vi "StringToHex.vi"(8 "error in (no error)":errorcluster caption="错误输入（无错误）", 11 "String_Hex":string="55AA001200050104110000000000000000000000000000000000000000000000") -> (0 "error out":errorcluster caption="错误输出", 2 "Hex":string)   [LabVIEW 2015]
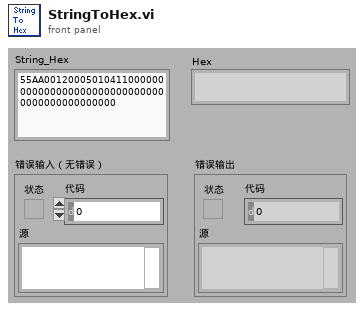
[diagram p1: front panel]
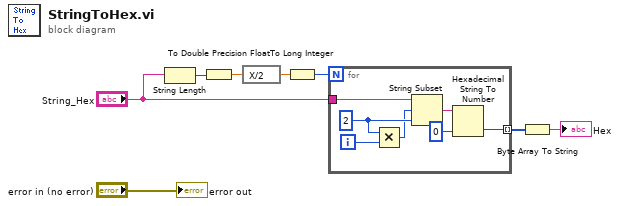
[diagram p0: block diagram]
diagram:
  n1 = String Length(string="String_Hex") -> (length=w8:i32)
  n2 = To Double Precision Float(number=w8) -> (double precision float=w7:dbl)
  n3 = expression code="X/2"(w7) -> (w6:dbl)
  n4 = To Long Integer(number=w6) -> (32bit integer=w5:i32)
  n5 = for {
    N: w5 -> [_]
    tunnel: "String_Hex" -> [w15]
    tunnel: [w10] -> w4 mode=indexing
    i -> [w14]
    w13 = 2 ("长度（剩余）")
    n6 = Multiply(x=w13, y=w14) -> (x*y=w12:i32)
    n7 = String Subset(string=w15, offset (0)=w12, length (rest)=w13) -> (substring=w9:string)
    n8 = Hexadecimal String To Number(string=w9, default (0uL)=u8 0 ("默认(0 U32)")) -> (number=w10:u8)  [unwired: 2 out]
  }
  n9 = Byte Array To String(unsigned byte array=w4) -> (string=→"Hex":string)
  "error out" <- "error in (no error)"
